vi "REG - Generate2DTest.vi"(8 "error in (no error)":errorcluster, 11 "Local":T5={"Parameters"={"Plot"=refnum, "Data"={"Split"={"X Train"=[], "X Test"=[], "Y Train"=[], "Y Test"=[]}, "Predict"=[]}, "Display"={"Choice"=enum."All", "Indexe"={"X"=0, "Y"=1}}, "Point Property"={"Train Style"=enum."Full circle", "Test OK Style"=enum."Full square", "Label Color"=[8978528, 4367871, 16716800], "Test NO OK"={"Style"=enum."Cross", "Color"=16711680}}, "Tolerance's threshold"=0.0}, "2D Array"=[], "Point ID"=[], "GoodPredict"=0, "Rating 2D Array"=[]}) -> (0 "error out":errorcluster, 3 "Local Out":T5={"Parameters"={"Plot"=refnum, "Data"={"Split"={"X Train"=[], "X Test"=[], "Y Train"=[], "Y Test"=[]}, "Predict"=[]}, "Display"={"Choice"=enum."All", "Indexe"={"X"=0, "Y"=1}}, "Point Property"={"Train Style"=enum."Full circle", "Test OK Style"=enum."Full square", "Label Color"=[8978528, 4367871, 16716800], "Test NO OK"={"Style"=enum."Cross", "Color"=16711680}}, "Tolerance's threshold"=0.0}, "2D Array"=[], "Point ID"=[], "GoodPredict"=0, "Rating 2D Array"=[]})   [LabVIEW 2020]
uses:
  _Controls/Datas.ctl
  _Controls/PointPropertyMultipleLabel.ctl
  _Controls/Style.ctl
  _Controls/2DData.ctl
types:
  T1 = typedef "Datas.ctl" = cluster{"Split":cluster{"X Train":dbl[][], "X Test":dbl[][], "Y Train":dbl[][], "Y Test":dbl[][]}, "Predict":dbl[][]}
  T2 = typedef "PointPropertyMultipleLabel.ctl" = cluster{"Train Style":T3, "Test OK Style":T3, "Label Color":u32[], "Test NO OK":cluster{"Style":T3, "Color":u32}}
  T3 = typedef "Style.ctl" = enum16{"Empty circle", "Full circle", "Empty square", "Full square", "Cross"}
  T4 = typedef "2DData.ctl" = cluster{"Tag":i32, "X":dbl[], "Y":dbl[]}
  T5 = cluster{"Parameters":cluster{"Plot":refnum<vi>, "Data":T1, "Display":cluster{"Choice":enum16{"All", "Train", "Test"}, "Indexe":cluster{"X":i32, "Y":i32}}, "Point Property":T2, "Tolerance's threshold":dbl}, "2D Array":cluster{"X":dbl[], "Y":dbl[]}[], "Point ID":cluster{"DataUse":enum16{"Dataset", "Train", "Test"}, "Color":u32}[], "GoodPredict":i32, "Rating 2D Array":T4[]}
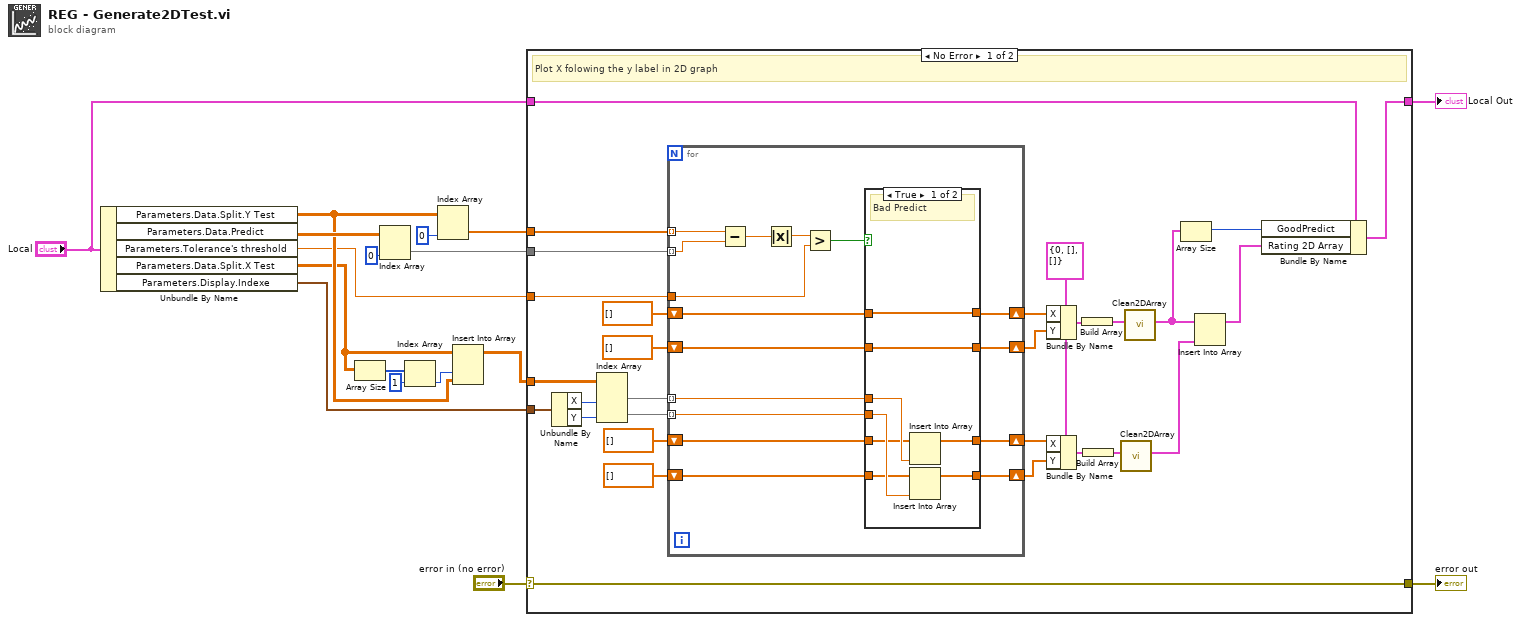
[diagram p0: block diagram]
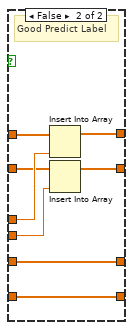
[diagram p2: hidden frame]
diagram:
  n1 = Unbundle By Name("Local") -> ("Parameters.Data.Split.Y Test"=w6:dbl[][], "Parameters.Data.Predict"=w14:dbl[][], "Parameters.Tolerance's threshold"=w1:dbl, "Parameters.Data.Split.X Test"=w5:dbl[][], "Parameters.Display.Indexe"=w9:cluster{"X":i32, "Y":i32})
  n2 = Array Size(array=w5) -> (size(s)=w3:i32[])
  n3 = Index Array(array=w14, index (col)=0 ("disabled index (col)")) -> (element=w12:dbl[])  [unwired: 1 in]
  n4 = Index Array(array=w3, index=1) -> (element=w4:i32)
  n5 = Index Array(array=w6, index (col)=0 ("disabled index (col)")) -> (element=w13:dbl[])  [unwired: 1 in]
  n6 = Insert Into Array(array=w5, index (col)=w4, new element=w6) -> (w7:dbl[][])  [unwired: 1 in]
  n7 = case shown="No Error" "error in (no error)" {
    selector: "error in (no error)" -> [w36 w80]
    tunnel: w7 -> [w44 _]
    tunnel: w12 -> [w19 _]
    tunnel: [w36 w80] -> w17
    tunnel: w13 -> [w20 _]
    tunnel: "Local" -> [w41 w79]
    tunnel: [w40 w79] -> w10
    tunnel: w9 -> [w38 _]
    tunnel: w1 -> [w18 _]
    frame No Error {
      w33 = T4 {"Tag"=0, "X"=[], "Y"=[]} ("2D Data")
      # "Plot X folowing the y label in 2D graph"
      n8 = Unbundle By Name(w38) -> ("X"=w43:i32, "Y"=w42:i32)
      n9 = Index Array(array=w44, index (col) #1=w43, index (col) #2=w42) -> (element #1=w46:dbl[], element #2=w45:dbl[])  [unwired: 2 in]
      n10 = for {
        tunnel: w46 -> [w61] mode=indexing
        tunnel: w45 -> [w62] mode=indexing
        tunnel: w19 -> [w47] mode=indexing
        tunnel: w20 -> [w48] mode=indexing
        shift-right: [w60] -> w32
        shift-left: dbl[] [] -> [w55]
        shift-right: [w59] -> w31
        shift-left: dbl[] [] -> [w56]
        shift-right: [w58] -> w30
        shift-left: dbl[] [] -> [w53]
        shift-right: [w57] -> w29
        shift-left: dbl[] [] -> [w54]
        tunnel: w18 -> [w51]
        n11 = Subtract(x=w48, y=w47) -> (x-y=w50:dbl)
        n12 = Absolute Value(x=w50) -> (abs(x)=w49:dbl)
        n13 = Greater?(x=w49, y=w51) -> (0:w52:bool)
        n14 = case shown="True" w52 {
          tunnel: w55 -> [w64 w78]
          tunnel: w61 -> [w70 w77]
          tunnel: [w64 w76] -> w60
          tunnel: [w65 w75] -> w59
          tunnel: w56 -> [w65 w74]
          tunnel: w62 -> [w69 w73]
          tunnel: w54 -> [w68 w71]
          tunnel: [w63 w71] -> w57
          tunnel: w53 -> [w67 w72]
          tunnel: [w66 w72] -> w58
          frame True {
            # "Bad Predict"
            n15 = Insert Into Array(array=w67, new element=w70) -> (w66:dbl[])  [unwired: 1 in]
            n16 = Insert Into Array(array=w68, new element=w69) -> (w63:dbl[])  [unwired: 1 in]
          }
          frame False {
            # "Good Predict Label"
            n17 = Insert Into Array(array=w78, new element=w77) -> (w76:dbl[])  [unwired: 1 in]
            n18 = Insert Into Array(array=w74, new element=w73) -> (w75:dbl[])  [unwired: 1 in]
          }
        }
      }
      n19 = Bundle By Name(cluster=w33, "X"=w32, "Y"=w31) -> (w28:T4)
      n20 = Bundle By Name(cluster=w33, "X"=w30, "Y"=w29) -> (w26:T4)
      n21 = Build Array(w28) -> (w27:T4[])
      n22 = Build Array(w26) -> (w25:T4[])
      n23 = call "Clean2DArray.vi"("Array2D"=w25) -> ("Array2DClean"=w34:T4[])  [unwired: 10 in]
      n24 = call "Clean2DArray.vi"("Array2D"=w27) -> ("Array2DClean"=w35:T4[])  [unwired: 10 in]
      n25 = Array Size(array=w35) -> (size(s)=w39:i32)
      n26 = Insert Into Array(array=w35, new element=w34) -> (w37:T4[])  [unwired: 1 in]
      n27 = Bundle By Name(cluster=w41, "GoodPredict"=w39, "Rating 2D Array"=w37) -> (w40:T5)
    }
    frame Error {
    }
  }
  "error out" <- w17
  "Local Out" <- w10
